vi "Save UI Attributes To Configuration.vi"(8 "error in (no error)":errorcluster, 10 "Selection Name":string, 11 "ScriptDialog in":refnum<class "ScriptDialog.lvclass">) -> (0 "error out":errorcluster, 3 "ScriptDialog out":refnum<class "ScriptDialog.lvclass">)   [LabVIEW 2015, in "ScriptDialog.lvclass"]
uses:
  ScriptDialog.lvclass
  ScriptDialog.lvclass/ScriptDialog.ctl
  System/UIConfiguration/UIConfiguration.lvclass
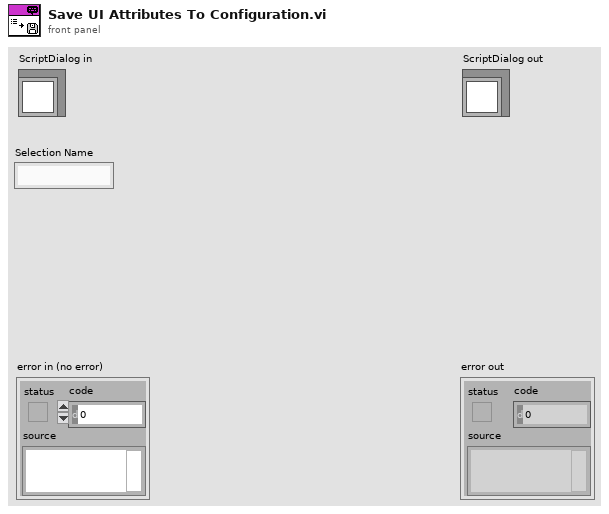
[diagram p1: front panel]
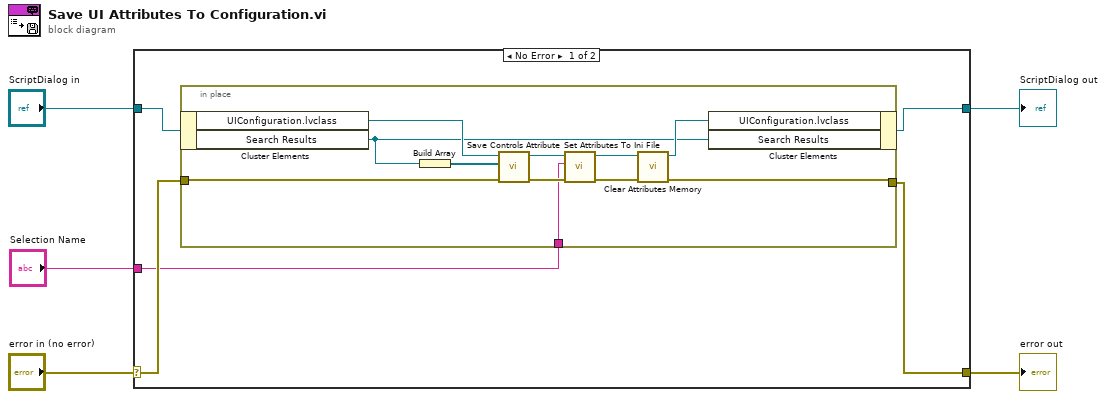
[diagram p0: block diagram]
diagram:
  n1 = case shown="No Error" "error in (no error)" {
    selector: "error in (no error)" -> [w10 w23]
    tunnel: [w6 w23] -> w4
    tunnel: [w7 w22] -> w2
    tunnel: "ScriptDialog in" -> [w8 w22]
    tunnel: "Selection Name" -> [w9 _]
    frame No Error {
      n2 = in-place {
        in-place-border: w10 -> [w16]
        in-place-border: w9 -> [w15]
        in-place-border: [w11] -> w6
        n3 = in-place-cluster #1(w8) -> ("UIConfiguration.lvclass"=w14:refnum<class "UIConfiguration.lvclass">, "Search Results"=w12:refnum<vi>)
        n4 = Build Array(w12) -> (w17:refnum<vi>[])
        n5 = call-dynamic "Save Controls Attribute.vi"("error in (no error)"=w16, "Control Refs"=w17, "UIConfiguration in"=w14) -> ("error out"=w20:errorcluster, "UIConfiguration out"=w21:refnum<class "UIConfiguration.lvclass">)  [unwired: 7 in]
        n6 = call "Set Attributes To Ini File.vi"("error in (no error)"=w20, "Selection Name"=w15, "UIConfiguration in"=w21) -> ("error out"=w18:errorcluster, "UIConfiguration out"=w19:refnum<class "UIConfiguration.lvclass">)  [unwired: 7 in]
        n7 = call "Clear Attributes Memory.vi"("error in (no error)"=w18, "UIConfiguration in"=w19) -> ("error out"=w11:errorcluster, "UIConfiguration out"=w13:refnum<class "UIConfiguration.lvclass">)  [unwired: 8 in]
        n8 = in-place-cluster #1("UIConfiguration.lvclass"=w13, "Search Results"=w12) -> (w7:refnum<class "ScriptDialog.lvclass">)
      }
    }
    frame Error {
    }
  }
  "error out" <- w4
  "ScriptDialog out" <- w2
